vi "Main.vi"() -> ()   [LabVIEW 2011]
uses:
  Expt_Device_Variable.ctl
  shared programs/MySQL/Preset Query Enum.ctl
  GUI_Template/GUI_master/tcp new data cluster.ctl
panel:
  out "replies":string[](array[string])
  in  "TCP collect timeout ms":i32=6000
  out "subarray":string[](array[string])
  out "expt devices":string[][](array[string])
  in  "Stop Button":bool
  in  "create new experiment":bool
  out "Expt Name":string
  out "Expt Device Array":string[](array[string])
  in  "Experiment":u16(ring) caption="Device Name" items=["Select Experiment to Copy", "10TW colliding pulse", "Bella", "FakeCam1only", "FakeCam1to5", "GOG", "Staging", "Staging cap alignment", "StagingTRA", "Test stand default", "TREX high power", "TREX low power"]
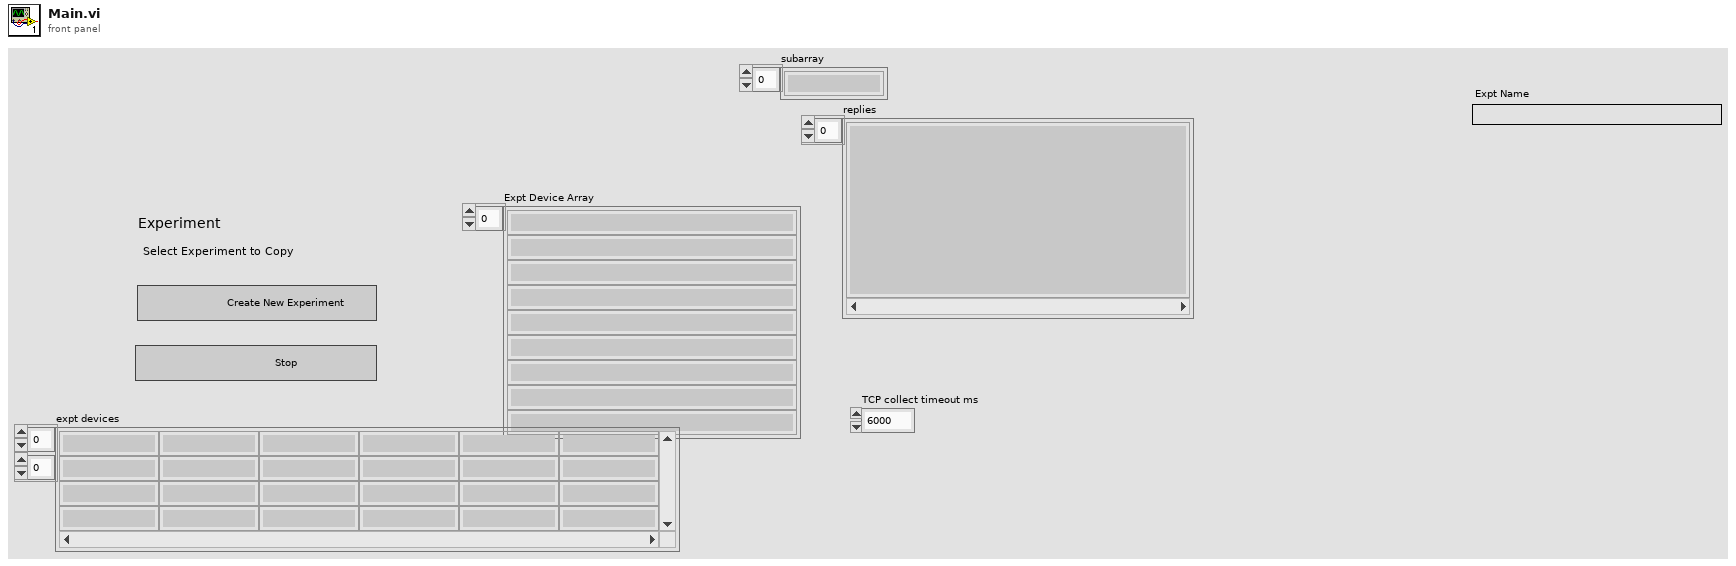
[diagram p1: front panel]
types:
  T1 = typedef "tcp new data cluster.ctl" = cluster{"EventEnum":enum16{"new data", "connection status update"}, "Device name":string}
  T2 = enum32{"invalid app kind", "Development System", "Run Time System", "Student Edition", "Embedded LabVIEW", "Evaluation", "Custom"}
  T3 = enum32{"Invalid", "Standard", "Closed", "Hidden", "Minimized", "Maximized"}
  T4 = typedef "Preset Query Enum.ctl" = enum16{"Get Locations", "Get all IPs and MACs", "Get classes", "Get expt variables to set at scanstart for particular device", "Get expt devices and variables with start values", "Get expt devices and variables (with data to get)", "Get expt devices with data to get", "Get Expt devices and GUIs", "Get all devices basic properties", "Get Virtual Devices Core Info", "Get Expt names", "Get experiment basic properties", "Get MC Ports", "Get device network comm port", "Get devicetype lvclass path", "Get basic device properties", "Get all setable variables of a device", "Get all variables of a devicetype", "Get all variables of a device", "Get all variables of device to save new experiment", "Get plotter details", "Get expt for plotter", "Get plotter IDs from expt", "Get all devices", "Get all Virtual Devices", "Get variable and device info for Virtual Device", "GetItemLocatorIP"}
  T5 = typedef "Expt_Device_Variable.ctl" = cluster{"Name":string, "Value":string, "Get":string, "Set":string, "Expt_dev_id":string, "Start Value":string, "End Value":string}
  T6 = cluster{"Core":cluster{"Current VI Reference":refnum<vi>, "Close Panel on Exit?":bool}, "Your Boolean data":bool, "Selected Experiment":string, "Experiment Names Array":string[], "Experiment Device Array":string[], "Expt_Device_Variables":T5[], "New Experiment Name":string, "TCP connection Array":refnum<k5>[]}
  T7 = cluster{"Current VI Reference":refnum<vi>, "Close Panel on Exit?":bool}
  T8 = typedef "mysql_authentication.ctl" = cluster{"User":string, "Password":string, "Database":string}
  T9 = cluster{"Port":u16, "IP Address":string, "Authentication":T8}
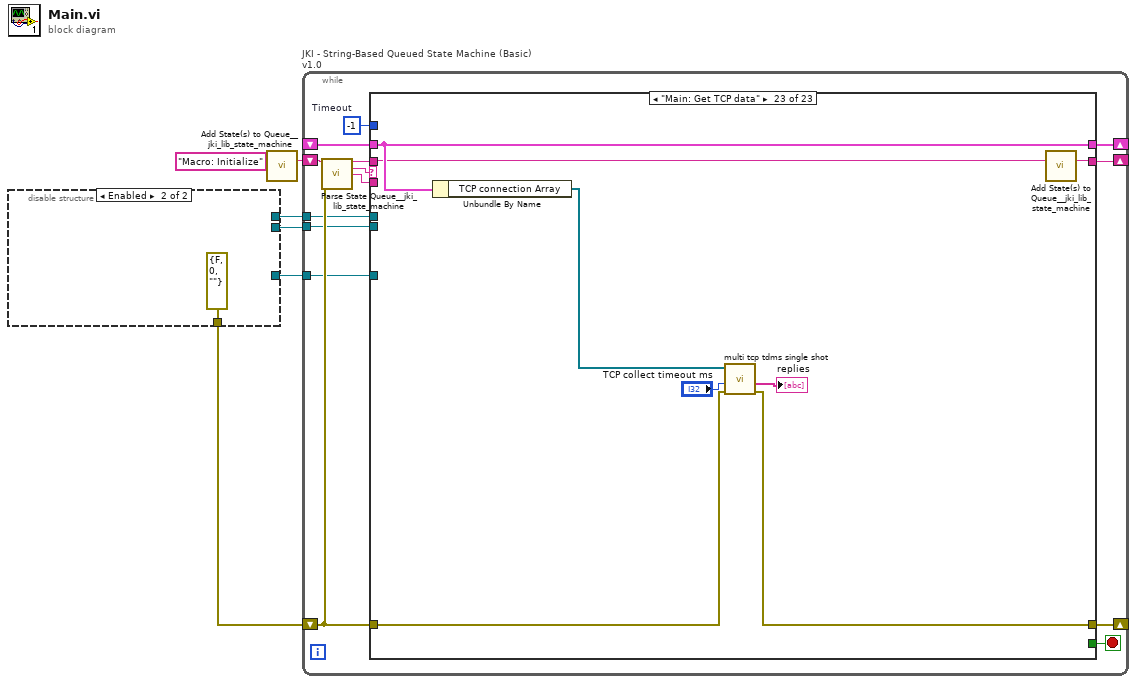
[diagram p0: block diagram]
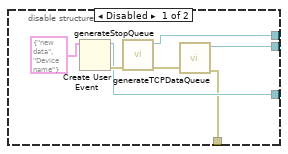
[diagram p2: hidden frame]
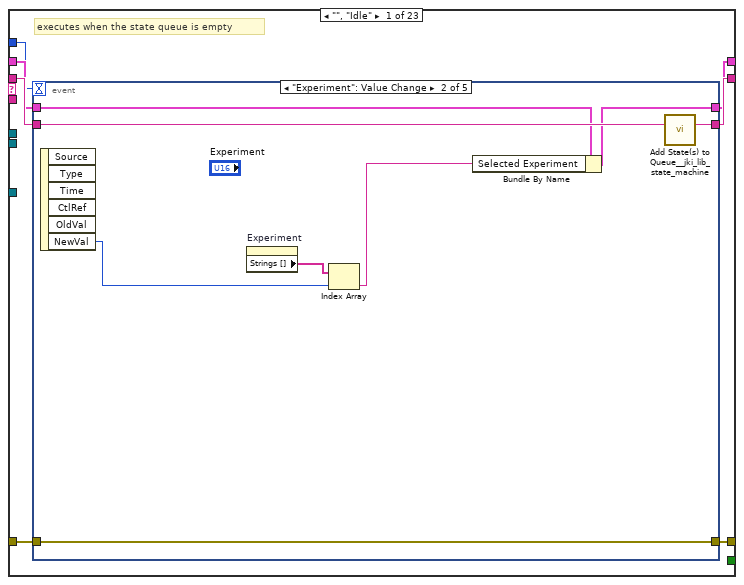
[diagram p3: hidden frame]
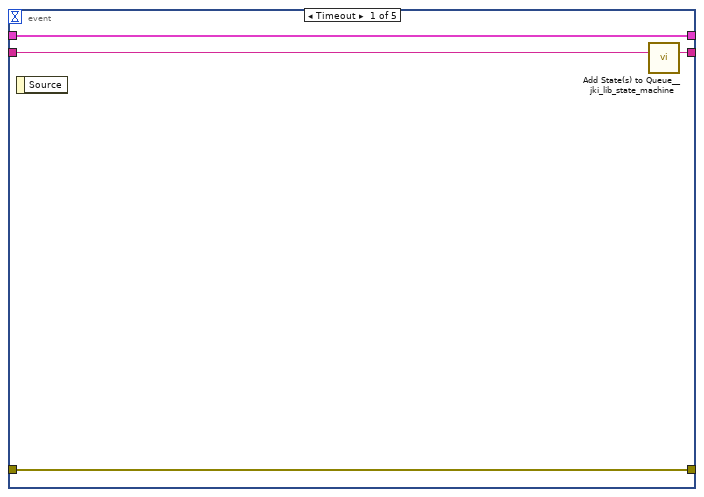
[diagram p4: hidden frame]
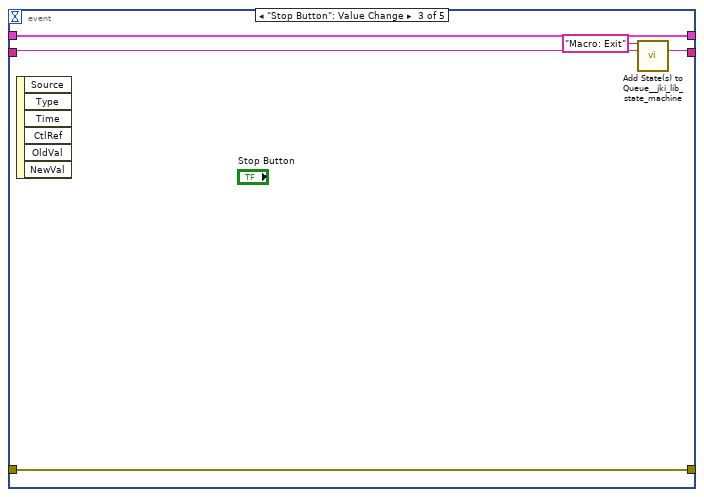
[diagram p5: hidden frame]
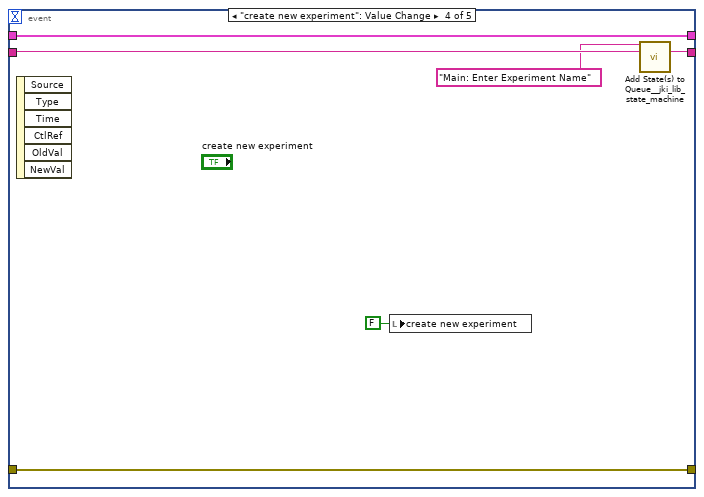
[diagram p6: hidden frame]
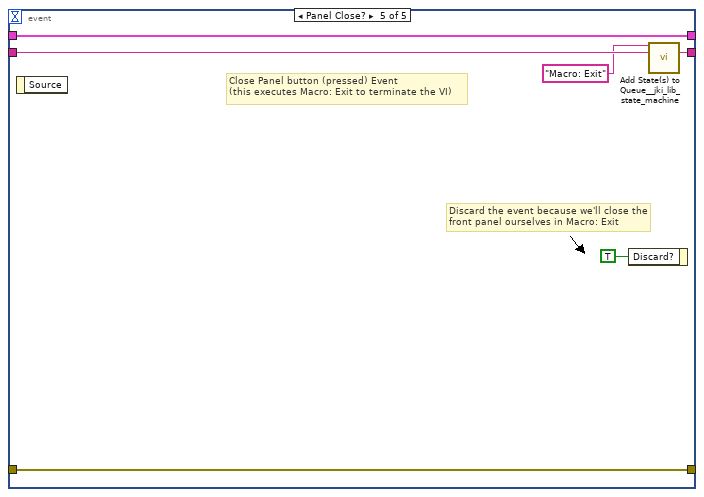
[diagram p7: hidden frame]
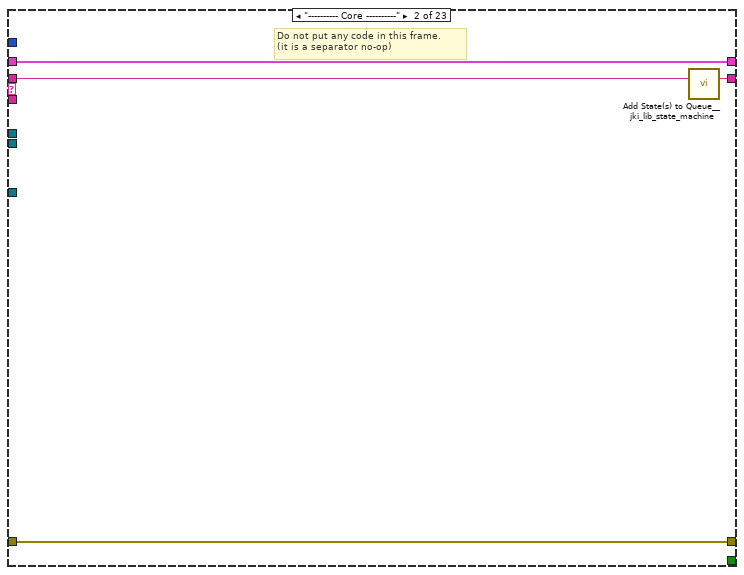
[diagram p8: hidden frame]
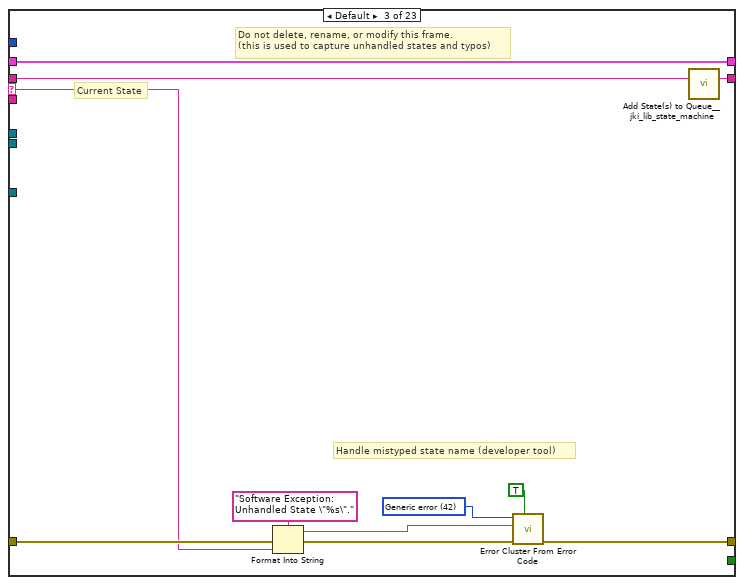
[diagram p9: hidden frame]
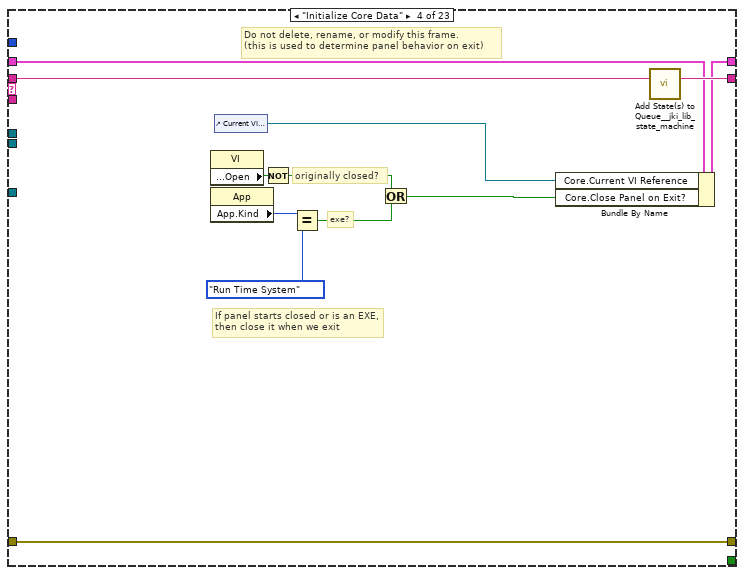
[diagram p10: hidden frame]
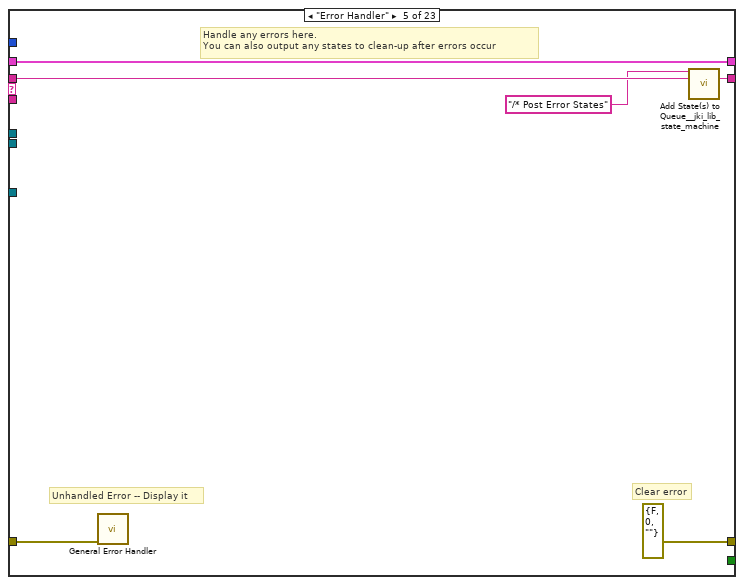
[diagram p11: hidden frame]
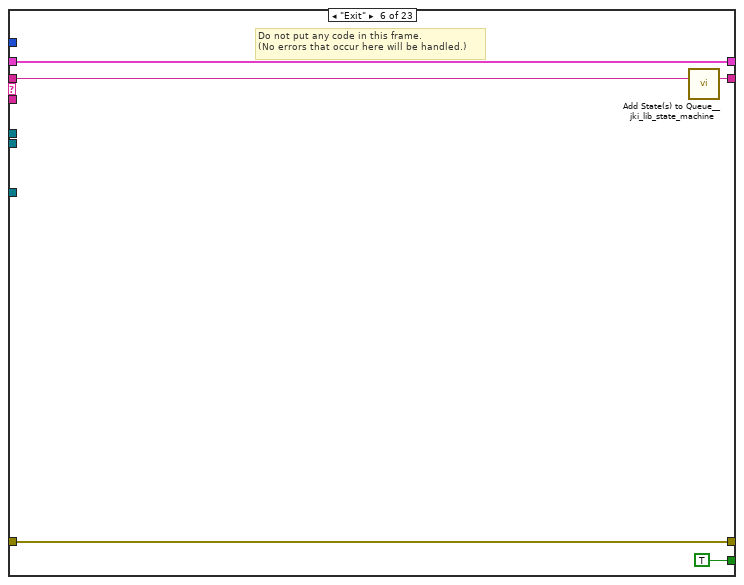
[diagram p12: hidden frame]
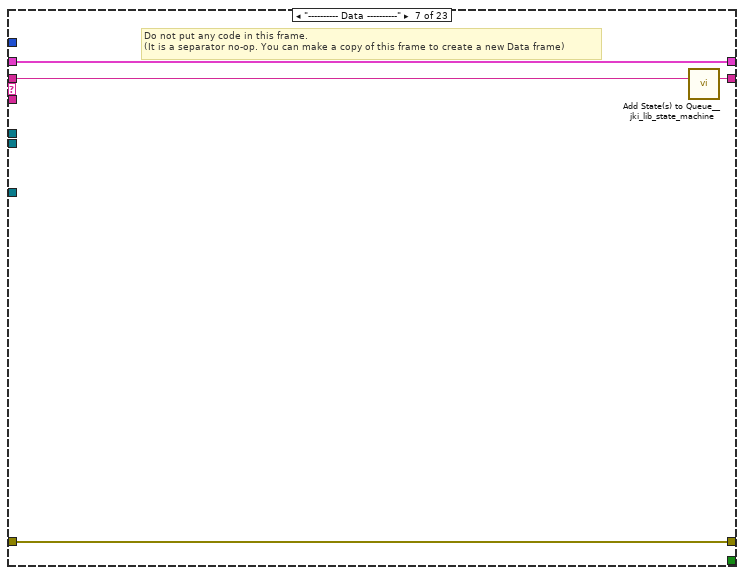
[diagram p13: hidden frame]
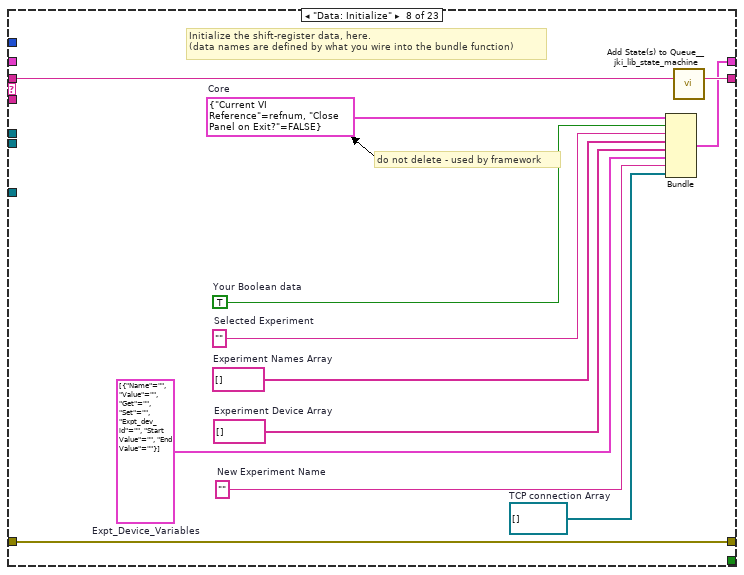
[diagram p14: hidden frame]
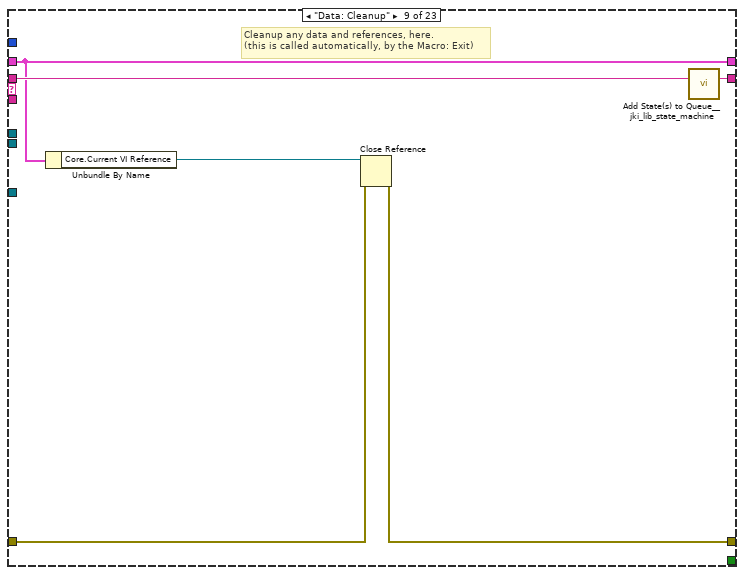
[diagram p15: hidden frame]
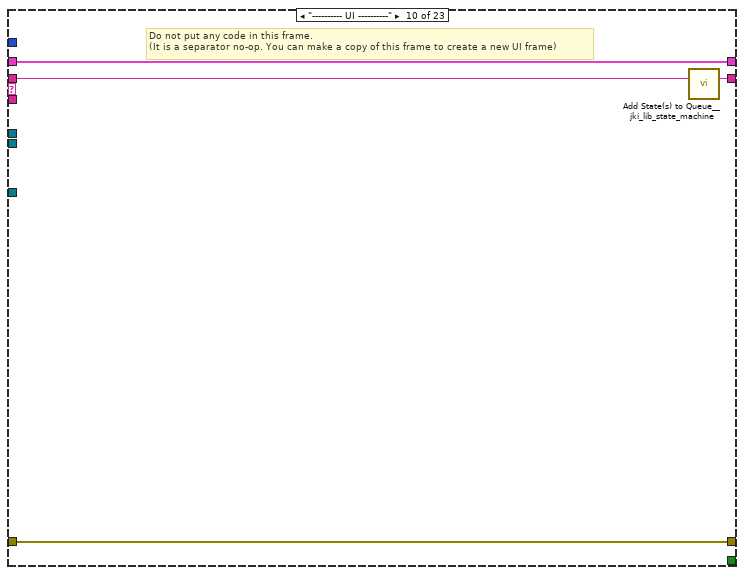
[diagram p16: hidden frame]
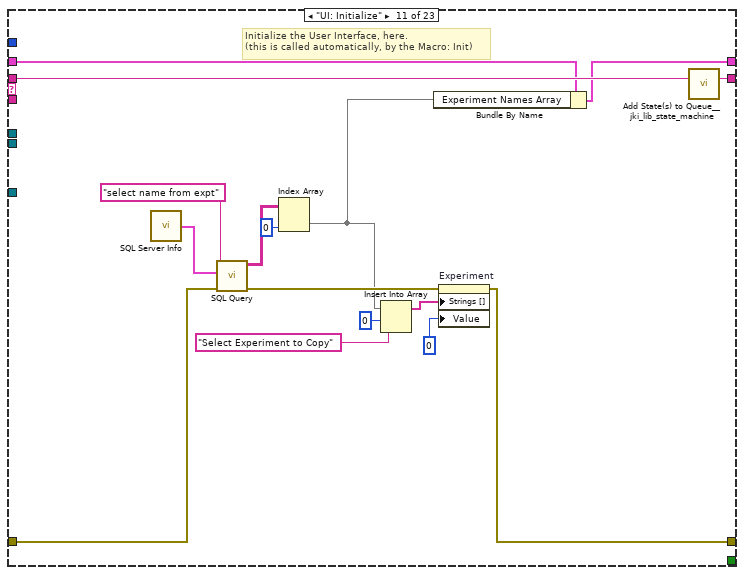
[diagram p17: hidden frame]
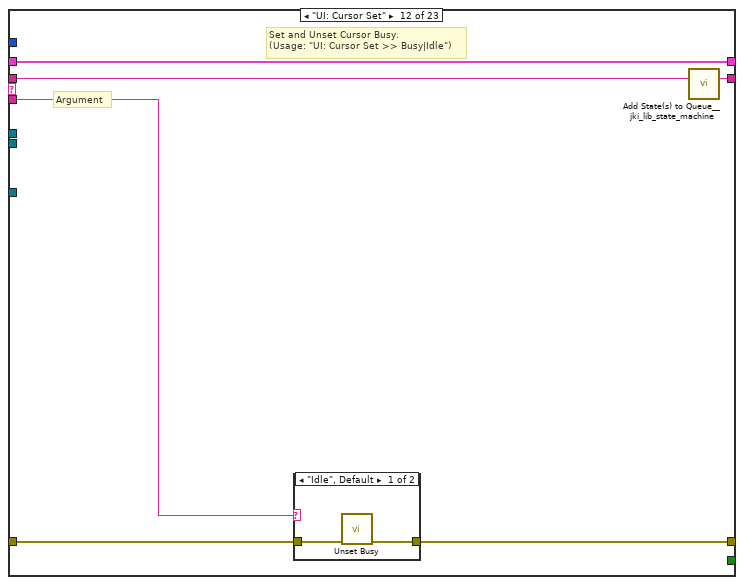
[diagram p18: hidden frame]
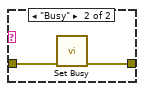
[diagram p19: hidden frame]
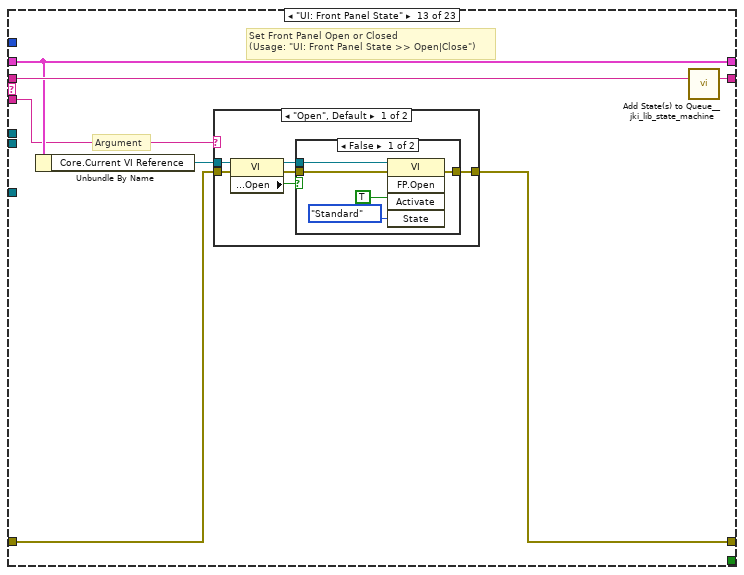
[diagram p20: hidden frame]
diagram:
  n1 = disable-structure shown="Enabled" {
    disable-tunnel: [w10 _] -> w4
    disable-tunnel: [w9 _] -> w3
    disable-tunnel: [w8 _] -> w2
    disable-tunnel: [w7 errorcluster {"status"=FALSE, "code"=0, "source"=""} ("error out")] -> w1
    frame Disabled {
      n2 = Create User Event(user event datatype=T1 {"EventEnum"=enum."new data", "Device name"="Device name"} ("New Event")) -> (user event=w10:refnum<user-event>, error out=w13:errorcluster)  [unwired: 1 in]
      n3 = call "generateStopQueue.vi"("error in (no error)"=w13) -> ("error out"=w12:errorcluster, "Queue out"=w9:refnum<queue>)  [unwired: 9 in]
      n4 = call "generateTCPDataQueue.vi"("error in (no error)"=w12) -> ("error out"=w7:errorcluster, "Queue out"=w8:refnum<queue>)  [unwired: 9 in]
    }
    frame Enabled {
    }
  }
  n5 = call <vilib>:"Add State(s) to Queue__jki_lib_state_machine.vi"("State(s) in (\"\")"="Macro: Initialize") -> ("States Out"=w6:string)  [unwired: 14 in]
  n6 = while "JKI - String-Based Queued State Machine (Basic) v1.0" {
    shift-right: [w21] -> _
    shift-left: _ -> [w20]
    shift-right: [w24] -> _
    shift-left: w1 -> [w18]
    shift-right: [w23] -> _
    shift-left: w6 -> [w25]
    tunnel: w4 -> [w17]
    tunnel: w3 -> [w16]
    tunnel: w2 -> [w15]
    stop <- w22 stop-if-true
    w19 = -1  # Timeout
    n7 = call <vilib>:"Parse State Queue__jki_lib_state_machine.vi"("State Queue"=w25, "Error In (no error)"=w18) -> ("Remaining States"=w27:string, "Current State"=w28:string, "Arguments"=w26:string)  [unwired: 11 in]
    n8 = case shown="\"Main: Get TCP data\"" w28 {
      selector: w28 -> [_ _ w69 _ _ _ _ _ _ _ _ _ _ _ _ _ _ _ _ _ _ _ _]
      tunnel: w27 -> [w35 w68 w73 w91 w97 w102 w106 w118 w124 w128 w144 w150 w161 w187 w192 w202 w206 w214 w232 w250 w269 w288 w316]
      tunnel: w26 -> [_ _ _ _ _ _ _ _ _ _ _ w145 w155 _ _ _ _ _ _ _ _ _ _]
      tunnel: w20 -> [w33 w65 w71 w82 w94 w100 w103 _ w119 w125 w137 w148 w157 w184 w189 w199 w203 w212 w234 w238 w261 w272 w318]
      tunnel: [w32 w66 w75 w88 errorcluster {"status"=FALSE, "code"=0, "source"=""} ("error out") w99 w104 w115 w120 w126 w130 w146 w158 w185 w190 w200 w204 w207 w229 w241 w257 w277 w319] -> w24
      tunnel: w18 -> [w31 w66 w74 w88 w93 w99 w104 w115 w121 w126 w131 w147 w159 w185 w190 w200 w204 w207 w230 w246 w258 w285 w320]
      tunnel: [w34 w67 w72 w90 w96 w101 w105 w117 w123 w127 w143 w149 w160 w186 w191 w201 w205 w215 w233 w251 w268 w287 w317] -> w23
      tunnel: [_ _ _ _ _ TRUE _ _ _ _ _ _ _ _ _ _ _ _ _ _ _ _ _] -> w22
      tunnel: [w30 w65 w71 w89 w94 w100 w103 w116 w119 w125 w136 w148 w157 w184 w189 w199 w203 w211 w234 w237 w260 w271 w318] -> w21
      tunnel: w19 -> [w29 _ _ _ _ _ _ _ _ _ _ _ _ _ _ _ _ _ _ _ _ _ _]
      tunnel: w17 -> [_ _ _ _ _ _ _ _ _ _ _ _ _ _ _ _ _ _ _ _ _ w281 _]
      tunnel: w16 -> [_ _ _ _ _ _ _ _ _ _ _ _ _ _ _ _ _ _ _ _ _ w280 _]
      tunnel: w15 -> [_ _ _ _ _ _ _ _ _ _ _ _ _ _ _ _ _ _ _ _ _ w279 _]
      frame "", "Idle" {
        # "executes when the state queue is empty"
        n9 = event shown="[1] \"Experiment\": Value Change" {
          selector: _ -> [_ _ _ _ _]
          dyn-events: _ -> [_ _ _ _ _]
          timeout: w29 -> [_ _ _ _ _]
          tunnel: w35 -> [w39 w46 w49 w54 w64]
          tunnel: [w38 w47 w50 w55 w63] -> w34
          tunnel: w33 -> [w36 w42 w51 w57 w61]
          tunnel: [w37 w45 w52 w56 w62] -> w32
          tunnel: w31 -> [w37 w45 w52 w56 w62]
          tunnel: [w36 w41 w51 w57 w61] -> w30
          event Timeout {
            n10 = event-data() -> ()  [unwired: 1 in, 1 out]
            n11 = call <vilib>:"Add State(s) to Queue__jki_lib_state_machine.vi"("State(s) in (\"\")"=w39) -> ("States Out"=w38:string)  [unwired: 14 in]
          }
          event "Experiment": Value Change {
            n12 = event-data() -> ("NewVal"=w43:u16)  [unwired: 1 in, 5 out]
            n13 = property on="Experiment" class="Ring (strict)"() -> ("Strings []"=w44:string[])  [unwired: 2 in, 2 out]
            n14 = Index Array(array=w44, index=w43) -> (element=w40:string)
            n15 = Bundle By Name(cluster=w42, "Selected Experiment"=w40) -> (w41:T6)
            n16 = call <vilib>:"Add State(s) to Queue__jki_lib_state_machine.vi"("State(s) in (\"\")"=w46) -> ("States Out"=w47:string)  [unwired: 14 in]
          }
          event "Stop Button": Value Change {
            n17 = event-data() -> ()  [unwired: 1 in, 6 out]
            n18 = call <vilib>:"Add State(s) to Queue__jki_lib_state_machine.vi"("State(s) in Front (\"\")"="Macro: Exit" ("State(s) in Front (\"\")"), "State(s) in (\"\")"=w49) -> ("States Out"=w50:string)  [unwired: 13 in]
          }
          event "create new experiment": Value Change {
            n19 = event-data() -> ()  [unwired: 1 in, 6 out]
            n20 = local write "create new experiment"(FALSE ("create new experiment")) -> ()
            n21 = call <vilib>:"Add State(s) to Queue__jki_lib_state_machine.vi"("State(s) in Front (\"\")"="Main: Enter Experiment Name" ("State(s) in Front (\"\")"), "State(s) in (\"\")"=w54) -> ("States Out"=w55:string)  [unwired: 13 in]
          }
          event Panel Close? {
            # "Discard the event because we'll close the front panel ourselves in Macro: Exit"
            # "Close Panel button (pressed) Event\n(this executes Macro: Exit to terminate the VI)"
            n22 = event-data() -> ()  [unwired: 1 in, 1 out]
            n23 = event-data("Discard?"=TRUE) -> ()  [unwired: 1 in, 1 out]
            n24 = call <vilib>:"Add State(s) to Queue__jki_lib_state_machine.vi"("State(s) in Front (\"\")"="Macro: Exit", "State(s) in (\"\")"=w64) -> ("States Out"=w63:string)  [unwired: 13 in]
          }
        }
      }
      frame "---------- Core ----------" {
        # "Do not put any code in this frame.\n(it is a separator no-op)"
        n25 = call <vilib>:"Add State(s) to Queue__jki_lib_state_machine.vi"("State(s) in (\"\")"=w68) -> ("States Out"=w67:string)  [unwired: 14 in]
      }
      frame Default {
        w78 = 42 items=["No error", "Argument error", "Memory is full", "Out of zone", "End of file", "File already open", "Generic file I/O error", "File not found", "File permission error", "Disk is full", "Duplicate path", "Too many files open", "System feature not enabled", "Resource file not found", "Cannot add resource", "Resource not found", "Image not found", "Image memory error", "Pen does not exist", "Config type invalid", "Config token not found", "Config parse error", "Config memory error", "Bad external code format", "Bad external code offset", "External code not present", "Null window", "Destroy window error", "Null menu", "Print aborted", "Bad print record", "Print driver error", "Windows error during printing", "Memory error during printing", "Print dialog error", "Generic print error", "Invalid device refnum", "Device not found", "Device parameter error", "Device unit error", "Cannot open device", "Device call aborted", "Generic error", "Cancelled by user", "Object ID too low", "Object ID too high", "Object not in heap", "Unknown heap", "Unknown object (invalid DefProc)", "Unknown object (DefProc not in table)", "Message out of range", "Invalid (null) method", "Unknown message", "Manager call not supported", "Bad address", "Network operation in progress", "Network operation timed out", "Connection is busy", "Network attribute not supported", "Network error", "Address in use", "System out of memory", "Connection aborted", "Connection refused", "Not connected", "Already connected", "Connection closed", "Initialization error (interapplication manager)", "Bad occurrence", "Wait on unbound occurrence handler", "Occurrence queue overflow", "Datalog type conflict", "Unused", "Unrecognized type (interapplication manager)", "Memory corrupt", "Failed to make temporary DLL", "Old CIN version", "Drag socket not found", "Failed to load drop-object", "Failed to register OLE object", "Failed to release OLE object", "Format specifier type mismatch", "Unknown format specifier", "Too few format specifiers", "Too many format specifiers", "Scan failed", "Newer CIN version", "Error converting to variant", "Runtime menu error", "Password tampered", "Variant attribute not found", "Incompatible variant data type", "Event data is not available", "Event Store is not present", "Occurrence is not found", "Event Queue is not created", "Event info is not available", "Refnum passed is NULL", "Error retrieving Class GUID", "Error retrieving CoClass GUID", "Error retrieving TypeLib GUID.", "Bad built application magic bytes.", "Specific driver is different from the specific driver associated with the Logical Name.", "There is no session opened to the class driver.", "Max Error", "MAX - Error with config objects", "MAX - Error loading configuration", "MAX - Group not supported"]
        # "Current State"
        # "Do not delete, rename, or modify this frame.\n(this is used to capture unhandled states and typos)"
        # "Handle mistyped state name (developer tool)"
        n26 = Format Into String(format string="Software Exception: Unhandled State \"%s\"." ("message"), error in=w74, w69) -> (resulting string=w77:string, error out=w76:errorcluster)  [unwired: 1 in]
        n27 = call <vilib>:"Error Cluster From Error Code.vi"("show call chain? (False)"=TRUE, "error in (no error)"=w76, "error message (\"\")"=w77, "error code (0)"=w78) -> ("error out"=w75:errorcluster)  [unwired: 5 in]
        n28 = call <vilib>:"Add State(s) to Queue__jki_lib_state_machine.vi"("State(s) in (\"\")"=w73) -> ("States Out"=w72:string)  [unwired: 14 in]
      }
      frame "Initialize Core Data" {
        # "Do not delete, rename, or modify this frame.\n(this is used to determine panel behavior on exit)"
        # "originally closed?"
        # "exe?"
        # "If panel starts closed or is an EXE, then close it when we exit"
        n29 = property class="VI"() -> ("Front Panel.Open"=w87:bool)  [unwired: 2 in, 2 out]
        n30 = property class="App"() -> ("App.Kind"=w86:T2)  [unwired: 2 in, 2 out]
        n31 = control-ref of="Current VI Reference"() -> (w80:refnum<vi>)
        n32 = Not(x=w87) -> (.not. x?=w84:bool)
        n33 = Equal?(x=w86, y=T2."Run Time System" ("Application:Kind")) -> (x = y?=w83:bool)
        n34 = Or(x=w84, y=w83) -> (x .or. y?=w81:bool)
        n35 = Bundle By Name(cluster=w82, "Core.Current VI Reference"=w80, "Core.Close Panel on Exit?"=w81) -> (w89:T6)
        n36 = call <vilib>:"Add State(s) to Queue__jki_lib_state_machine.vi"("State(s) in (\"\")"=w91) -> ("States Out"=w90:string)  [unwired: 14 in]
      }
      frame "Error Handler" {
        # "Unhandled Error -- Display it"
        # "Handle any errors here.\nYou can also output any states to clean-up after errors occur"
        # "Clear error"
        n37 = call <vilib>:"General Error Handler.vi"("error in (no error)"=w93) -> ()  [unwired: 10 in, 5 out]
        n38 = call <vilib>:"Add State(s) to Queue__jki_lib_state_machine.vi"("State(s) in Front (\"\")"="/* Post Error States", "State(s) in (\"\")"=w97) -> ("States Out"=w96:string)  [unwired: 13 in]
      }
      frame "Exit" {
        # "Do not put any code in this frame.\n(No errors that occur here will be handled.)"
        n39 = call <vilib>:"Add State(s) to Queue__jki_lib_state_machine.vi"("State(s) in (\"\")"=w102) -> ("States Out"=w101:string)  [unwired: 14 in]
      }
      frame "---------- Data ----------" {
        # "Do not put any code in this frame.\n(It is a separator no-op. You can make a copy of this frame to create a new Data frame)"
        n40 = call <vilib>:"Add State(s) to Queue__jki_lib_state_machine.vi"("State(s) in (\"\")"=w106) -> ("States Out"=w105:string)  [unwired: 14 in]
      }
      frame "Data: Initialize" {
        w107 = refnum<k5>[] []  # TCP connection Array
        w108 = ""  # New Experiment Name
        w109 = T5[] [{"Name"="", "Value"="", "Get"="", "Set"="", "Expt_dev_id"="", "Start Value"="", "End Value"=""}]  # Expt_Device_Variables
        w110 = string[] []  # Experiment Device Array
        w111 = string[] []  # Experiment Names Array
        w112 = T7 {"Current VI Reference"=refnum, "Close Panel on Exit?"=FALSE}  # Core
        w114 = TRUE  # Your Boolean data
        w113 = ""  # Selected Experiment
        # "do not delete - used by framework"
        # "Initialize the shift-register data, here.\n(data names are defined by what you wire into the bundle function)"
        n41 = Bundle("Core"=w112, "Your Boolean data"=w114, "Selected Experiment"=w113, "Experiment Names Array"=w111, "Experiment Device Array"=w110, "Expt_Device_Variables"=w109, "New Experiment Name"=w108, "TCP connection Array"=w107) -> (w116:T6)  [unwired: 1 in]
        n42 = call <vilib>:"Add State(s) to Queue__jki_lib_state_machine.vi"("State(s) in (\"\")"=w118) -> ("States Out"=w117:string)  [unwired: 14 in]
      }
      frame "Data: Cleanup" {
        # "Cleanup any data and references, here.\n(this is called automatically, by the Macro: Exit)"
        n43 = Unbundle By Name(w119) -> ("Core.Current VI Reference"=w122:refnum<vi>)
        n44 = Close Reference(reference=w122, error in (no error)=w121) -> (error out=w120:errorcluster)
        n45 = call <vilib>:"Add State(s) to Queue__jki_lib_state_machine.vi"("State(s) in (\"\")"=w124) -> ("States Out"=w123:string)  [unwired: 14 in]
      }
      frame "---------- UI ----------" {
        # "Do not put any code in this frame.\n(It is a separator no-op. You can make a copy of this frame to create a new UI frame)"
        n46 = call <vilib>:"Add State(s) to Queue__jki_lib_state_machine.vi"("State(s) in (\"\")"=w128) -> ("States Out"=w127:string)  [unwired: 14 in]
      }
      frame "UI: Initialize" {
        # "Initialize the User Interface, here.\n(this is called automatically, by the Macro: Init)"
        n47 = call "SQL Server Info.vi"() -> ("SQL Server Info"=w142:T9)
        n48 = call "SQL Query.vi"("error in (no error)"=w131, "SQL Server Info"=w142, "Query"="select name from expt") -> ("error out"=w138:errorcluster, "data"=w140:string[][])  [unwired: 7 in]
        n49 = Index Array(array=w140, index (col)=0 ("disabled index (col)")) -> (element=w135:string[])  [unwired: 1 in]
        n50 = Insert Into Array(array=w135, index=0, new element="Select Experiment to Copy" ("new element/subarray")) -> (w132:string[])
        n51 = Bundle By Name(cluster=w137, "Experiment Names Array"=w135) -> (w136:T6)
        n52 = property on="Experiment" class="Ring (strict)"(error in=w138, "Strings []"=w132, "Value"=0) -> (error out=w130:errorcluster)  [unwired: 1 in, 1 out]
        n53 = call <vilib>:"Add State(s) to Queue__jki_lib_state_machine.vi"("State(s) in (\"\")"=w144) -> ("States Out"=w143:string)  [unwired: 14 in]
      }
      frame "UI: Cursor Set" {
        # "Argument"
        # "Set and Unset Cursor Busy.\n(Usage: \"UI: Cursor Set >> Busy|Idle\")"
        n54 = case shown="\"Idle\", Default" w145 {
          tunnel: w147 -> [w152 w154]
          tunnel: [w151 w153] -> w146
          frame "Idle", Default {
            n55 = call <vilib>:"Unset Busy.vi"("error in (no error)"=w152) -> ("error out"=w151:errorcluster)  [unwired: 10 in]
          }
          frame "Busy" {
            n56 = call <vilib>:"Set Busy.vi"("error in (no error)"=w154) -> ("error out"=w153:errorcluster)  [unwired: 9 in, 1 out]
          }
        }
        n57 = call <vilib>:"Add State(s) to Queue__jki_lib_state_machine.vi"("State(s) in (\"\")"=w150) -> ("States Out"=w149:string)  [unwired: 14 in]
      }
      frame "UI: Front Panel State" {
        # "Argument"
        # "Set Front Panel Open or Closed\n(Usage: \"UI: Front Panel State >> Open|Close\")"
        n58 = Unbundle By Name(w157) -> ("Core.Current VI Reference"=w156:refnum<vi>)
        n59 = case shown="\"Open\", Default" w155 {
          tunnel: w159 -> [w165 w178]
          tunnel: [w167 w179] -> w158
          tunnel: w156 -> [w166 w176]
          frame "Open", Default {
            n60 = property class="VI"(reference=w166, error in=w165) -> (reference out=w163:refnum<vi>, error out=w164:errorcluster, "Front Panel.Open"=w162:bool)
            n61 = case shown="False" w162 {
              tunnel: [w170 w173] -> w167
              tunnel: w164 -> [w169 w173]
              tunnel: w163 -> [w168 _]
              frame False {
                n62 = invoke class="VI" method="FP.Open"(reference=w168, error in=w169, "Activate"=TRUE, "State"=T3."Standard") -> (error out=w170:errorcluster)  [unwired: 1 in, 4 out]
              }
              frame True {
              }
            }
          }
          frame "Close" {
            n63 = property class="VI"(reference=w176, error in=w178) -> (reference out=w175:refnum<vi>, error out=w177:errorcluster, "Front Panel.Open"=w174:bool)
            n64 = case shown="True" w174 {
              tunnel: [w180 w183] -> w179
              tunnel: w177 -> [w180 w182]
              tunnel: w175 -> [_ w181]
              frame False {
              }
              frame True {
                n65 = invoke class="VI" method="FP.Close"(reference=w181, error in=w182) -> (error out=w183:errorcluster)  [unwired: 1 in, 2 out]
              }
            }
          }
        }
        n66 = call <vilib>:"Add State(s) to Queue__jki_lib_state_machine.vi"("State(s) in (\"\")"=w161) -> ("States Out"=w160:string)  [unwired: 14 in]
      }
      frame "---------- Macro ----------" {
        # "Do not put any code in this frame.\n(It is a separator no-op. You can make a copy of this frame to create a new Macro frame)"
        n67 = call <vilib>:"Add State(s) to Queue__jki_lib_state_machine.vi"("State(s) in (\"\")"=w187) -> ("States Out"=w186:string)  [unwired: 14 in]
      }
      frame "Macro: Initialize" {
        w188 = "Data: Initialize\nInitialize Core Data\nUI: Initialize\nUI: Front Panel State >> Open"  # Data: Initialize Initialize Core Data UI: Initialize UI: Front Panel State >> Open
        # "Initialization Macro\n(This is called once, when the VI starts)"
        n68 = call <vilib>:"Add State(s) to Queue__jki_lib_state_machine.vi"("State(s) in Front (\"\")"=w188, "State(s) in (\"\")"=w192) -> ("States Out"=w191:string)  [unwired: 13 in]
      }
      frame "Macro: Exit" {
        # "Exit Macro\n(This is called once, when the VI exits)"
        n69 = Unbundle By Name(w199) -> ("Core.Close Panel on Exit?"=w198:bool)
        n70 = Select(t="UI: Front Panel State >> Close", s=w198, f="") -> (s? t:f=w195:string)
        n71 = call <vilib>:"Add State(s) to Queue__jki_lib_state_machine.vi"("State(s) in (\"\")"=w195, "State(s) at Back (\"\")"="Data: Cleanup\nExit") -> ("States Out"=w193:string)  [unwired: 13 in]
        n72 = call <vilib>:"Add State(s) to Queue__jki_lib_state_machine.vi"("State(s) in Front (\"\")"=w193, "State(s) in (\"\")"=w202) -> ("States Out"=w201:string)  [unwired: 13 in]
      }
      frame "---------- Main ----------" {
        # "Template Separator\n(You can make a copy of, or modify, this frame)"
        n73 = call <vilib>:"Add State(s) to Queue__jki_lib_state_machine.vi"("State(s) in (\"\")"=w206) -> ("States Out"=w205:string)  [unwired: 14 in]
      }
      frame "Main: Enter Experiment Name" {
        n74 = call "Enter Experiment Name"() -> ("Expt Name"=w213:string, "OK"=w210:bool)  [unwired: 17 in, 1 out]
        n75 = case shown="True" w210 {
          tunnel: w213 -> [_ w220]
          tunnel: ["" w222] -> w209
          tunnel: ["" w219] -> w208
          frame False {
          }
          frame True {
            n76 = Empty String/Path?(string/path=w220) -> (empty?=w221:bool)
            n77 = Select(t="", s=w221, f=w220) -> (s? t:f=w219:string)
            n78 = Select(t="", s=w221, f="Main: Add New Experiment to DB") -> (s? t:f=w222:string)
            "Expt Name" <- w220
          }
        }
        n79 = Bundle By Name(cluster=w212, "New Experiment Name"=w208) -> (w211:T6)
        n80 = call <vilib>:"Add State(s) to Queue__jki_lib_state_machine.vi"("State(s) in Front (\"\")"=w209, "State(s) in (\"\")"=w214) -> ("States Out"=w215:string)  [unwired: 13 in]
      }
      frame "Main: Add New Experiment to DB" {
        n81 = Unbundle By Name(w234) -> ("New Experiment Name"=w231:string)
        n82 = call "AddExperiment.vi"("error in (no error)"=w230, "Experiment Name"=w231) -> ("error out"=w229:errorcluster, "Quit ?"=w228:bool)  [unwired: 1 in]
        n83 = Select(t="", s=w228, f="Main: Add Experiment Devices to DB" ("t")) -> (s? t:f=w227:string)
        n84 = call <vilib>:"Add State(s) to Queue__jki_lib_state_machine.vi"("State(s) in Front (\"\")"=w227, "State(s) in (\"\")"=w232) -> ("States Out"=w233:string)  [unwired: 13 in]
      }
      frame "Main: Add Experiment Devices to DB" {
        n85 = Unbundle By Name(w238) -> ("New Experiment Name"=w243:string, "Selected Experiment"=w245:string)
        n86 = call "SQL Server Info.vi"() -> ("SQL Server Info"=w247:T9)
        n87 = Concatenate Strings("select device,GUIexe, GUI_IP, GUIscreenx, GUIscreeny,enabled from expt_device where expt='" ("Query"), w245, "' AND enabled='yes'" ("string")) -> (w249:string)
        n88 = call "SQL Query.vi"("error in (no error)"=w246, "SQL Server Info"=w247, "Query"=w249) -> ("error out"=w242:errorcluster, "data"=w240:string[][])  [unwired: 7 in]
        "expt devices" <- w240
        n89 = Index Array(array=w240, index (col)=0 ("disabled index (col)")) -> (element=w236:string[])  [unwired: 1 in]
        n90 = Bundle By Name(cluster=w238, "Experiment Device Array"=w236) -> (w237:T6)
        n91 = for {
          tunnel: w240 -> [w254] mode=indexing
          tunnel: w243 -> [w255]
          tunnel: w242 -> [w253]
          tunnel: [w252] -> w241
          n92 = call "Add Expt Device.vi"("error in (no error)"=w253, "Expt Device Details"=w254, "Experiment Name"=w255) -> ("error out"=w252:errorcluster)  [unwired: 8 in]
        }
        n93 = call <vilib>:"Add State(s) to Queue__jki_lib_state_machine.vi"("State(s) in Front (\"\")"="Main: Get Experiment Device Variables" ("State(s) in Front (\"\")"), "State(s) in (\"\")"=w250) -> ("States Out"=w251:string)  [unwired: 13 in]
      }
      frame "Main: Get Experiment Device" {
        # "THIS CASE NOT BEING CURRENTLY USED. DELETE LATER\nIF USED LATER, DELETE THIS MSG"
        n94 = Unbundle By Name(w261) -> ("Selected Experiment"=w262:string)
        n95 = call "preset SQL Queries.vi"("error in (no error)"=w258, "Expt name / MCIP/ Variable Name"=w262, "Preset Query"=Preset_Query_Enum."Get Expt devices and GUIs") -> ("error out"=w257:errorcluster, "data"=w263:string[][])  [unwired: 6 in, 1 out]
        n96 = Delete From Array(array=w263, index (row)=0) -> (array with subset deleted=w266:string[][])  [unwired: 2 in, 1 out]
        n97 = Index Array(array=w266, index (col)=0 ("disabled index (col)")) -> (element=w259:string[])  [unwired: 1 in]
        "Expt Device Array" <- w259
        n98 = Bundle By Name(cluster=w261, "Experiment Device Array"=w259) -> (w260:T6)
        n99 = call <vilib>:"Add State(s) to Queue__jki_lib_state_machine.vi"("State(s) in Front (\"\")"="Main: Get Experiment Device Variables" ("State(s) in Front (\"\")"), "State(s) in (\"\")"=w269) -> ("States Out"=w268:string)  [unwired: 13 in]
      }
      frame "Main: Get Experiment Device Variables" {
        # "Your code here.\n(You can make a copy of, or modify, this frame)"
        n100 = Unbundle By Name(w272) -> ("Experiment Device Array"=w282:string[], "Selected Experiment"=w286:string)
        n101 = for {
          tunnel: w286 -> [w314]
          tunnel: w285 -> [w313]
          tunnel: [w312] -> w278
          tunnel: w282 -> [w311] mode=indexing
          tunnel: [w307] -> w275 mode=indexing
          n102 = call "preset SQL Queries.vi"("error in (no error)"=w313, "Expt name / MCIP/ Variable Name"=w314, "Device/Devicetype name\n/Plotter.id/#"=w311, "Preset Query"=Preset_Query_Enum."Get all setable variables of a device") -> ("error out"=w312:errorcluster, "data"=w310:string[][])  [unwired: 5 in, 1 out]
          n103 = Index Array(array=w310, index (col)=0 ("disabled index (col)")) -> (element=w308:string[])  [unwired: 1 in]
          "subarray" <- w308
          n104 = call "parse subscribe command.vi"("variable names"=w308) -> ("Subscribe command"=w307:string)  [unwired: 6 in]
        }
        n105 = call "preset SQL Queries.vi"("Preset Query"=Preset_Query_Enum."Get all devices basic properties") -> ("data"=w284:string[][])  [unwired: 8 in, 2 out]
        n106 = call "get info from core device data.vi"("devices to get data from"=w282, "All Devices Core Info"=w284) -> ("Ports"=w274:string[], "IP Addresses"=w276:string[])  [unwired: 2 in]
        n107 = disable-structure shown="Enabled" {
          disable-tunnel: w281 -> [w297 _]
          disable-tunnel: w280 -> [w296 _]
          disable-tunnel: w279 -> [w295 _]
          disable-tunnel: w278 -> [w294 w300]
          disable-tunnel: [w293 w299] -> w277
          disable-tunnel: w276 -> [w291 w304]
          disable-tunnel: w275 -> [w290 w302]
          disable-tunnel: w274 -> [w289 w303]
          disable-tunnel: [_ w298] -> w270
          frame Disabled {
            n108 = call "build tcp initialize message for process vis.vi"("IP Addresses"=w291, "Ports"=w289, "Subscribe commands"=w290) -> ("subscribe messages\nfor process vis"=w292:string[])  [unwired: 8 in]
            n109 = call "reentrant tcp data get sub vi.vi"("tcp data event"=w297, "error in (no error)"=w294, "tcpDataqueue"=w295, "Stopqueue"=w296, "subscribe messages for process vis"=w292) -> ("error out"=w293:errorcluster)  [unwired: 6 in]
          }
          frame Enabled {
            n110 = call "TCP multiple open.vi"("timeout ms (60000)"=1000, "Ports"=w303, "error in 1 (no error)"=w300, "IP Addresses"=w304) -> ("error out"=w301:errorcluster, "Array"=w298:refnum<k5>[])  [unwired: 1 out]
            n111 = call "tcp multiple write.vi"("Connection ID array"=w298, "error in 1 (no error)"=w301, "messages to send"=w302, "timeout ms (25000)"=1000) -> ("error out"=w299:errorcluster)
          }
        }
        n112 = Bundle By Name(cluster=w272, "TCP connection Array"=w270) -> (w271:T6)
        n113 = call <vilib>:"Add State(s) to Queue__jki_lib_state_machine.vi"("State(s) in Front (\"\")"="Main: Get TCP data" ("State(s) in Front (\"\")"), "State(s) in (\"\")"=w288) -> ("States Out"=w287:string)  [unwired: 13 in]
      }
      frame "Main: Get TCP data" {
        n114 = Unbundle By Name(w318) -> ("TCP connection Array"=w322:refnum<k5>[])
        n115 = call "multi tcp tdms single shot.vi"("TCP connections"=w322, "timeout ms"="TCP collect timeout ms", "error in"=w320) -> ("replies"=→"replies":string[], "error out"=w319:errorcluster)  [unwired: 2 in, 2 out]
        n116 = call <vilib>:"Add State(s) to Queue__jki_lib_state_machine.vi"("State(s) in (\"\")"=w316) -> ("States Out"=w317:string)  [unwired: 14 in]
      }
    }
  }
